vi "FP RT main.vi"() -> ()   [LabVIEW 2014]
uses:
  <vilib>/userdefined/High Color/IMAQdx.ctl
  <vilib>/myRIO/Instrument Drivers/Onboard IO/PWM/typedefs/PWM Reference.ctl
  <vilib>/myRIO/Common/Instrument Driver Framework/Utilities/typedefs/myRIO Generic Hardware Reference.ctl
  <vilib>/myRIO/Common/Instrument Driver Framework/Utilities/typedefs/Hardware Version Enum.ctl
  <vilib>/myRIO/Common/Instrument Driver Framework/Utilities/typedefs/myRIO v1.0 Reference.ctl
  <vilib>/myRIO/Common/Instrument Driver Framework/Utilities/typedefs/Generic FPGA Reference.ctl
  <vilib>/myRIO/Common/Instrument Driver Framework/myRIO v1.0/PWM/typedefs/PWM Channels Enum.ctl
  <vilib>/myRIO/Instrument Drivers/Onboard IO/PWM/typedefs/PWM Configuration.ctl
  <vilib>/userdefined/High Color/nirio_resource_hc.ctl
  <vilib>/myRIO/Instrument Drivers/Onboard IO/DIO/typedefs/DIO Reference.ctl
  <vilib>/myRIO/Common/Instrument Driver Framework/myRIO v1.0/DIO/typedefs/DIO Channels List.ctl
  <vilib>/myRIO/Common/Instrument Driver Framework/myRIO v1.0/DIO/typedefs/DIO Channels Enum.ctl
  <vilib>/myRIO/Instrument Drivers/Onboard IO/AI/typedefs/AI Reference.ctl
  <vilib>/myRIO/Common/Instrument Driver Framework/myRIO v1.0/AI/typedefs/AI Channels List.ctl
  <vilib>/myRIO/Common/Instrument Driver Framework/myRIO v1.0/AI/typedefs/AI Channels Enum.ctl
  <vilib>/myRIO/Common/Instrument Driver Framework/Utilities/typedefs/Analog Scaling Constants List.ctl
  <vilib>/myRIO/Common/Instrument Driver Framework/Utilities/typedefs/Analog Scaling Constants.ctl
  <vilib>/myRIO/Common/Instrument Driver Framework/myRIO v1.0/PWM/vis/myRIO v1.1 Open PWM.vi
  <vilib>/myRIO/Common/Instrument Driver Framework/myRIO v1.0/DIO/vis/myRIO v1.1 Open DIO.vi
  <vilib>/myRIO/Common/Instrument Driver Framework/myRIO v1.0/AI/vis/myRIO v1.1 Open AI.vi
  <vilib>/myRIO/Common/Instrument Driver Framework/Utilities/vis/Validate Channels.vi
  <vilib>/myRIO/Common/Instrument Driver Framework/myRIO v1.0/PWM/vis/myRIO v1.0 Reserve PWM.vi
  <vilib>/myRIO/Common/Instrument Driver Framework/myRIO v1.0/DIO/vis/myRIO v1.0 Reserve DIO.vi
  <vilib>/myRIO/Common/Instrument Driver Framework/myRIO v1.0/AI/vis/myRIO v1.0 Reserve AI.vi
  <vilib>/myRIO/Common/Instrument Driver Framework/myRIO v1.0/PWM/vis/myRIO v1.0 Build MUX Configuration PWM.vi
  <vilib>/myRIO/Common/Instrument Driver Framework/myRIO v1.0/Resource Manager/vis/myRIO v1.0 Reserve Channel List.vi
  <vilib>/myRIO/Common/Instrument Driver Framework/myRIO v1.0/DIO/vis/myRIO v1.0 Build MUX Configuration DIO.vi
  <vilib>/myRIO/Common/Instrument Driver Framework/myRIO v1.0/AI/vis/myRIO v1.0 Build MUX Configuration AI.vi
  <vilib>/myRIO/Common/Instrument Driver Framework/myRIO v1.0/Resource Manager/vis/myRIO v1.0 Create Configuration List.vi
  <vilib>/myRIO/Common/Instrument Driver Framework/myRIO v1.0/Resource Manager/vis/myRIO v1.0 Reserve Channel.vi
  <vilib>/myRIO/Common/Instrument Driver Framework/myRIO v1.0/Resource Manager/vis/myRIO v1.0 Unreserve Channel.vi
  <vilib>/myRIO/Common/Instrument Driver Framework/myRIO v1.0/Resource Manager/vis/myRIO v1.0 Build Mutex Name.vi
  <vilib>/Utility/VariantDataType/GetNumericInfo.vi
  <vilib>/Utility/error.llb/Error Cluster From Error Code.vi
  <vilib>/myRIO/Common/Instrument Driver Framework/myRIO v1.0/myRIO v1.1 Open.vi
  <vilib>/myRIO/Common/Instrument Driver Framework/myRIO v1.0/AI/vis/myRIO v1.0 Get Scaling Constants AI.vi
  <vilib>/myRIO/Common/Instrument Driver Framework/Utilities/vis/IO Manager.vi
  <vilib>/myRIO/Common/Instrument Driver Framework/Utilities/vis/Configuration Manager.vi
  <vilib>/myRIO/Common/Instrument Driver Framework/myRIO v1.0/myRIO v1.0 Close.vi
  <vilib>/myRIO/Common/Instrument Driver Framework/myRIO v1.0/Resource Manager/vis/myRIO v1.0 Configure IO.vi
  <vilib>/myRIO/Instrument Drivers/Onboard IO/AI/vis/myRIO AI Open.xnode
  <vilib>/myRIO/Instrument Drivers/Onboard IO/DIO/vis/myRIO DIO Open.xnode
  <vilib>/myRIO/Instrument Drivers/Onboard IO/PWM/vis/myRIO PWM Open.xnode
  <vilib>/vision/driver/NI_Vision_Acquisition_Software.lvlib
  <vilib>/myRIO/Instrument Drivers/Onboard IO/AI/AI.lvlib
  <vilib>/myRIO/Instrument Drivers/Onboard IO/DIO/DIO.lvlib
  <vilib>/myRIO/Instrument Drivers/Onboard IO/PWM/PWM.lvlib
panel:
  in  "Tab Control":T1(tab)
  out "GLED":bool
  out "BLED":bool
  out "RLED":bool
  out "BW Image":T2(plugin-control)
  in  "stop":bool
  out "Midbrain?":bool
  out "Rudder":dbl(knob) min=-45.0 max=45.0 step=1.0 scale=-45.0..45.0
  out "Speed":dbl(knob) min=-9.0 max=9.0 step=1.0 scale=-50.0..50.0
  out "Hindbrain?":bool
  out "Forebrain?":bool
  out "Battery Dead?":bool
  out "Complete?":bool=TRUE
  out "Arbiter Graph":cluster{dbl, dbl, dbl[]}(graph)
  in  "Session In":T3="cam0"
  out "Color Image":T2(plugin-control)
  out "Nb Circles":i32
  out "UDP Time Out?":bool
  in  "Tug letter":string="G"
  in  "Run?":bool
  in  "MSpeed":dbl(slide) scale=-50.0..50.0 scale format="%#.1g"
  in  "MHeading":dbl(slide) scale=-180.0..180.0 scale format="%_1f"
  in  "Manual?":bool
  out "Camera Data":T4(array[cluster])
  out "Boat Status":T5={"GPS"={"X pos"=0, "Y pos"=0, "Heading"=0.0}, "IR Sensors"=[{"Name"="Bow", "Angle"=0.0, "Distance"=0.0}], "MOT BAT"=7.2, "RIO BAT"=7.2}
  out "GPS?":bool
  out "Act Com":T6
  out "Forebrain ACT":dbl[](array[numeric])
  out "IR Sensors":T7(array[cluster])
  out "GPS":cluster{"X pos":i32, "Y pos":i32, "Heading":dbl}
  out "RED LED":bool
  out "GREEN LED":bool
  out "BLUE LED":bool
  in  "MDF":T8(array[cluster])=[{"Type"=enum."Start", "X"=250, "Y"=250, "Speed"=0, "Behaviors"=enum."Open Water Transit"}, {"Type"=enum."Waypoint", "X"=400, "Y"=100, "Speed"=20, "Behaviors"=enum."P-Wall Follow"}, {"Type"=enum."Waypoint", "X"=250, "Y"=250, "Speed"=20, "Behaviors"=enum."Open Water Transit"}, {"Type"=enum."Waypoint", "X"=250, "Y"=400, "Speed"=20, "Behaviors"=enum."Open Water Transit"}, {"Type"=enum."Waypoint", "X"=100, "Y"=400, "Speed"=20, "Behaviors"=enum."Open Water Transit"}, {"Type"=enum."End", "X"=250, "Y"=250, "Speed"=0, "Behaviors"=enum."Open Water Transit"}]
  out "Invalid Pos?":bool
  out "error out":errorcluster
  out "Forebrain Comd":T9
  out "Debug IR \nRaw Readings":T7(array[cluster])
  out "size(s)":i32
  out "MDF Active":T8(array[cluster])
  # "BEHAVIOR LIGHTS"
  # "To start the Tug, press the \">\" key in the tool bar.\n\nPress the Run? control to start the Mission.\n\nWhen complete the Complete? indicator will light.\n\nIf the Run? is not pressed again, the mission will start again.\n\nAlways press the STOP button to end the operation!!!!!!!!!!!!!"
  # "Press the Manual? button to control\nthe Tug from the sliders"
  # "Stuck indicates that\nthe boat is not moving."
  # "Enter the Letter\nof  your Tug"
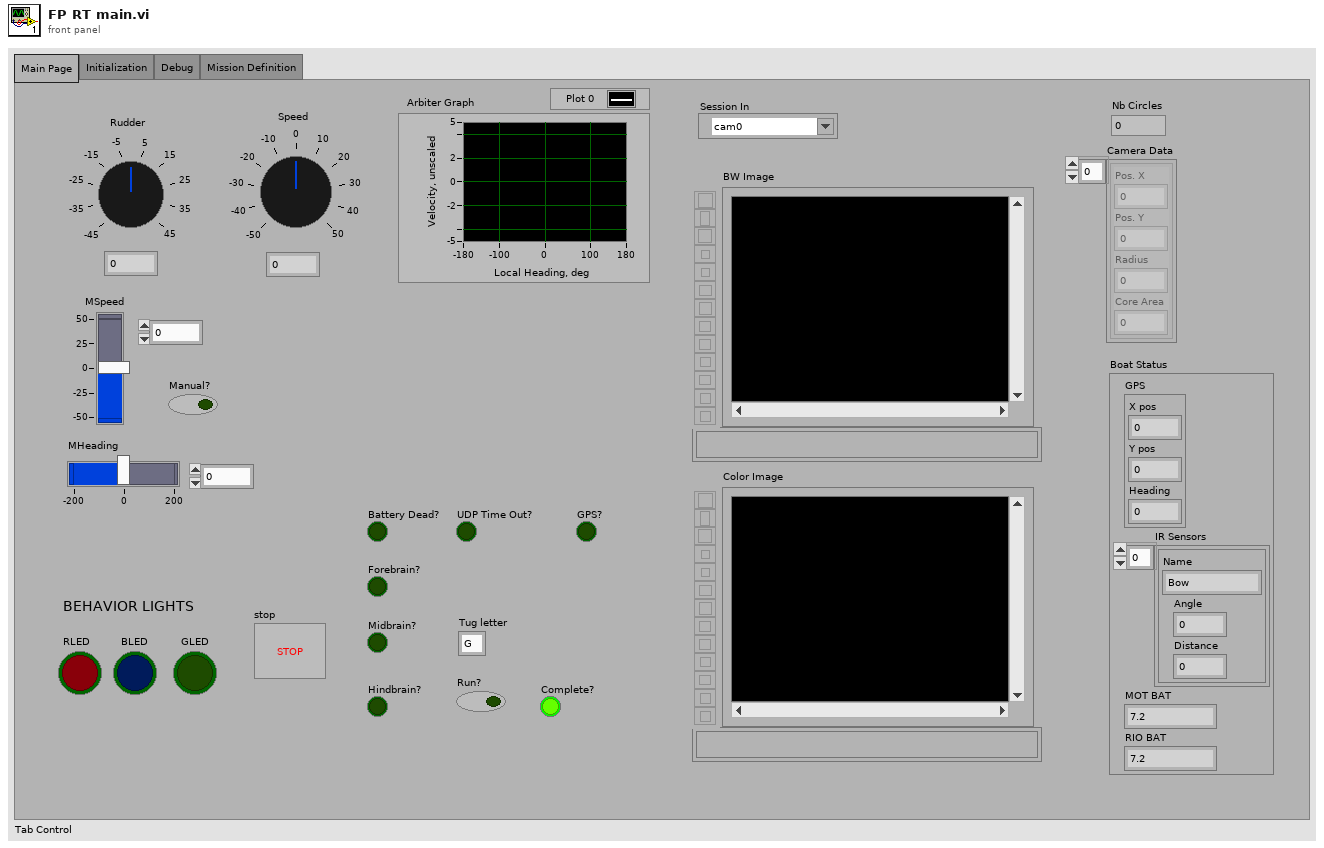
[diagram p1: front panel]
types:
  T1 = enum32{"Main Page", "Initialization", "Debug", "Mission Definition"}
  T2 = typedef "IMAQ Image.ctl" = refnum<image>
  T3 = typedef "IMAQdx.ctl" = refnum<k21>
  T4 = cluster{"Pos. X":i32, "Pos. Y":i32, "Radius":i32, "Core Area":i32}[]
  T5 = cluster{"GPS":cluster{"X pos":i32, "Y pos":i32, "Heading":dbl}, "IR Sensors":cluster{"Name":string, "Angle":dbl, "Distance":dbl}[], "MOT BAT":dbl, "RIO BAT":dbl}
  T6 = cluster{"Desired Local\nHeading":dbl, "Desired\nSpeed":dbl}
  T7 = cluster{"Name":string, "Angle":dbl, "Distance":dbl}[]
  T8 = cluster{"Type":enum16{"Start", "Waypoint", "End"}, "X":i32, "Y":i32, "Speed":i32, "Behaviors":enum16{"Open Water Transit", "P-Wall Follow", "S-Wall Follow", "Dock"}}[]
  T9 = cluster{"Behaviors":enum16{"Open Water Transit", "P-Wall Follow", "S-Wall Follow", "Dock"}, "Behavior\nVelocity":dbl}
  T10 = typedef "nirio_resource_hc.ctl" = tag
  T11 = typedef "Hardware Version Enum.ctl" = enum16{"Unknown", "myRIO-1900", "myRIO-1950"}
  T12 = typedef "Image Type" = u32
  T13 = enum16{"Open Water Transit", "P-Wall Follow", "S-Wall Follow", "Dock"}
  T14 = typedef "PWM.lvlib/PWM Reference.ctl" = cluster{"myRIO Reference":T15, "PWM Channels Enum":T18, "PWM Configuration":T19}
  T15 = typedef "myRIO Generic Hardware Reference.ctl" = cluster{"myRIO Model":T11, "myRIO Hardware Reference":T16}
  T16 = typedef "myRIO v1.0 Reference.ctl" = cluster{"Generic FPGA Reference":T17, "Allow multiple opens":bool}
  T17 = typedef "Generic FPGA Reference.ctl" = refnum<k20>
  T18 = typedef "PWM Channels Enum.ctl" = enum16{"Not Connected", "C/PWM0", "C/PWM1", "A/PWM0", "A/PWM1", "A/PWM2", "B/PWM0", "B/PWM1", "B/PWM2"}
  T19 = typedef "PWM.lvlib/PWM Configuration.ctl" = cluster{"Frequency":dbl, "Duty Cycle":dbl}
  T20 = typedef "DIO.lvlib/DIO Reference.ctl" = cluster{"myRIO Reference":T15, "DIO Channels List":T21}
  T21 = typedef "DIO Channels List.ctl" = T22[]
  T22 = typedef "DIO Channels Enum.ctl" = enum16{"Not Connected", "C/DIO0", "C/DIO1", "C/DIO2", "C/DIO3", "C/DIO4", "C/DIO5", "C/DIO6", "C/DIO7", "A/DIO0", "A/DIO1", "A/DIO2", "A/DIO3", "A/DIO4", "A/DIO5", "A/DIO6", "A/DIO7", "A/DIO8", "A/DIO9", "A/DIO10", "A/DIO11", "A/DIO12", "A/DIO13", "A/DIO14", "A/DIO15", "B/DIO0", "B/DIO1", "B/DIO2", "B/DIO3", "B/DIO4", "B/DIO5", "B/DIO6", "B/DIO7", "B/DIO8", "B/DIO9", "B/DIO10", "B/DIO11", "B/DIO12", "B/DIO13", "B/DIO14", "B/DIO15", "LED0", "LED1", "LED2", "LED3", "Button0"}
  T23 = typedef "AI.lvlib/AI Reference.ctl" = cluster{"myRIO Reference":T15, "AI Channels List":T24, "AI Scaling Constants List":T26}
  T24 = typedef "AI Channels List.ctl" = T25[]
  T25 = typedef "AI Channels Enum.ctl" = enum16{"Not Connected", "AudioIn/Left", "AudioIn/Right", "C/AI0", "C/AI1", "A/AI0", "A/AI1", "A/AI2", "A/AI3", "B/AI0", "B/AI1", "B/AI2", "B/AI3"}
  T26 = typedef "Analog Scaling Constants List.ctl" = T27[]
  T27 = typedef "Analog Scaling Constants.ctl" = cluster{"LSB Weight (Volts)":dbl, "Offset (Volts)":dbl, "Signed?":bool}
  T28 = cluster{"Obs Avoid Array":dbl[], "P-Wall Array":dbl[], "S-Wall Array":dbl[], "Unstuck Array":dbl[]}
  T29 = cluster{"regular expression":string, i32, i32, i32}
  T30 = cluster{"Behaviors":enum16{"Open Water Transit", "P-Wall Follow", "S-Wall Follow", "Dock"}, dbl}
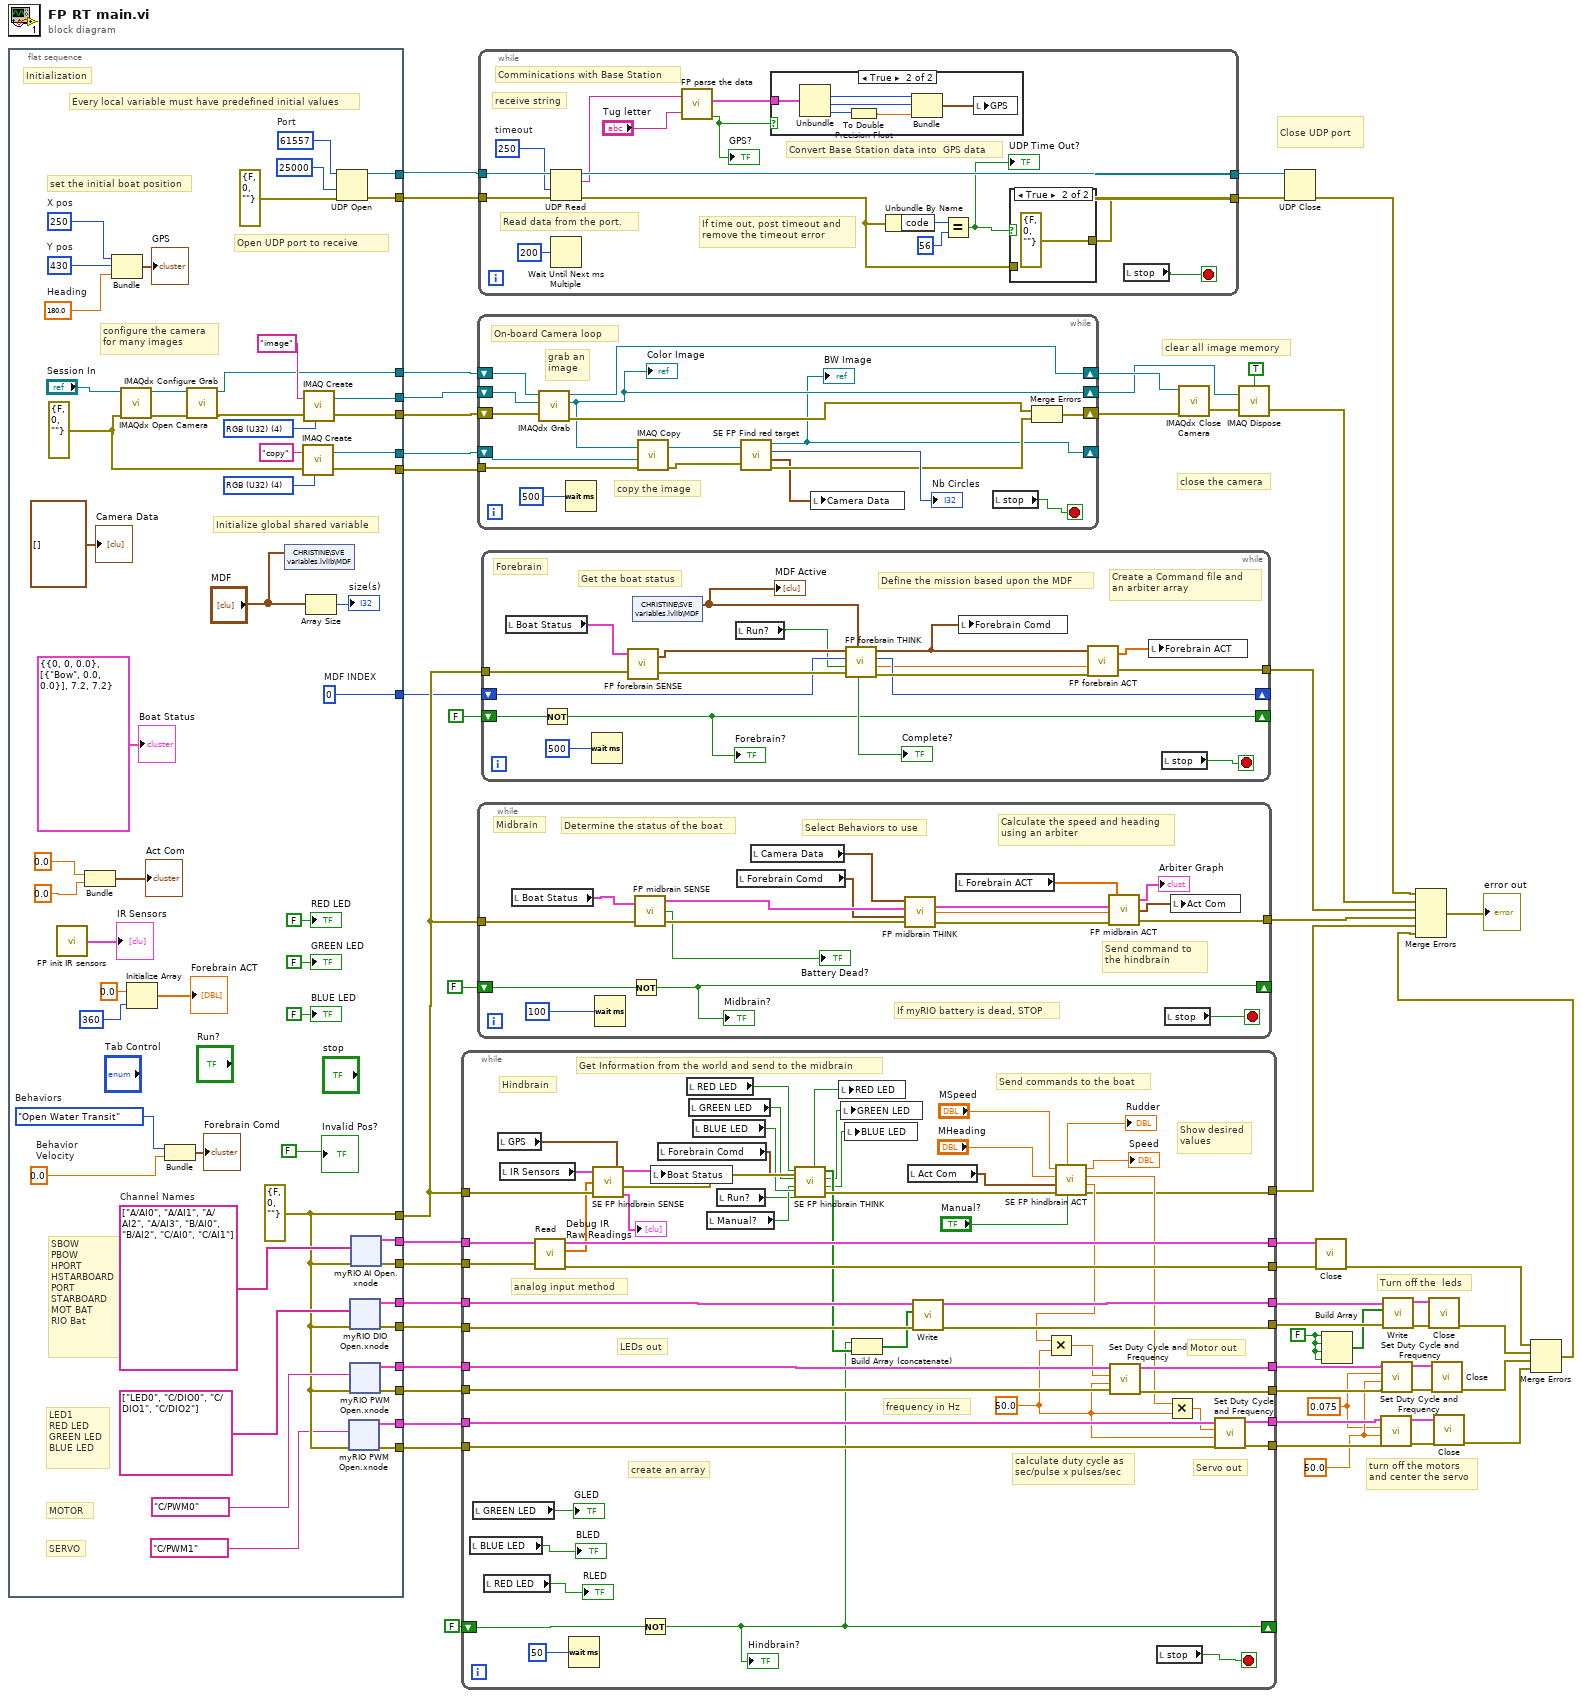
[diagram p0: block diagram]
diagram:
  w2 = 0.075
  w1 = FALSE
  w3 = 50.0
  # "Turn off the  leds"
  # "turn off the motors\nand center the servo"
  # "Close UDP port"
  # "clear all image memory"
  # "close the camera"
  n1 = flat-sequence {
    tunnel: [w68] -> w51
    tunnel: [w103] -> w48
    tunnel: [w94] -> w47
    tunnel: [w93] -> w46
    tunnel: [w92] -> w45
    tunnel: [w88] -> w38
    tunnel: [w87] -> w39
    tunnel: [w83] -> w33
    tunnel: [w82] -> w34
    tunnel: [w76] -> w31
    tunnel: [w75] -> w30
    tunnel: [w73] -> w26
    tunnel: [w72] -> w27
    tunnel: [w70] -> w25
    tunnel: [w69] -> w24
    tunnel: [w66] -> w23
    tunnel: [w65] -> w22
    frame #0 {
      w77 = tag[] ["A/AI0", "A/AI1", "A/AI2", "A/AI3", "B/AI0", "B/AI2", "C/AI0", "C/AI1"]  # Channel Names
      w79 = 430  # Y pos
      w80 = 250  # X pos
      w81 = 180.0  # Heading
      w86 = u16 61557  # Port
      w91 = T12 4 items=["Grayscale (U8)", "Grayscale (I16)", "Grayscale (SGL)", "Complex (CSG)", "RGB (U32)", "HSL (U32)", "RGB (U64)", "Grayscale (U16)"] ("Image Type")
      w89 = errorcluster {"status"=FALSE, "code"=0, "source"=""} ("error in")
      w99 = T12 4 items=["Grayscale (U8)", "Grayscale (I16)", "Grayscale (SGL)", "Complex (CSG)", "RGB (U32)", "HSL (U32)", "RGB (U64)", "Grayscale (U16)"] ("Image Type")
      w68 = errorcluster {"status"=FALSE, "code"=0, "source"=""} ("error out")
      w103 = 0  # MDF INDEX
      w107 = 0.0  # Behavior Velocity
      w102 = T13."Open Water Transit"  # Behaviors
      # "Initialize global shared variable"
      # "LED1\nRED LED\nGREEN LED\nBLUE LED"
      # "SERVO"
      # "MOTOR"
      # "SBOW\nPBOW\nHPORT\nHSTARBOARD\nPORT\nSTARBOARD\nMOT BAT\nRIO Bat"
      # "set the initial boat position"
      # "Open UDP port to receive"
      # "configure the camera\nfor many images"
      # "Every local variable must have predefined initial values"
      # "Initialization"
      n2 = call "FP init IR sensors.vi"() -> ("IR Sensors"=→"IR Sensors":T7)  [unwired: 1 in]
      n3 = Bundle(0.0, 0.0) -> (→"Act Com":cluster{dbl, dbl})  [unwired: 1 in]
      n4 = Bundle("X pos"=w80, "Y pos"=w79, "Heading"=w81) -> (→"GPS":cluster{"X pos":i32, "Y pos":i32, "Heading":dbl})  [unwired: 1 in]
      n5 = call <vilib>:"IMAQdx Open Camera.vi"("error in"=w89, "Session In"="Session In") -> ("error out"=w96:errorcluster, "Session Out"=w95:T3)  [unwired: 1 in, 7 out]
      n6 = Initialize Array(0.0 ("element"), 360 ("dimension size")) -> (→"Forebrain ACT":dbl[])
      n7 = Bundle("Behaviors"=w102, "Behavior\nVelocity"=w107) -> (→"Forebrain Comd":T9)  [unwired: 1 in]
      n8 = call <vilib>:"IMAQdx Configure Grab.vi"("error in"=w96, "Session In"=w95) -> ("error out"=w100:errorcluster, "Session Out"=w92:T3)  [unwired: 8 out]
      n9 = shared-variable "CHRISTINE\\SVE variables.lvlib\\MDF"("MDF") -> ()  [unwired: 1 in, 1 out]
      n10 = call "IMAQ Create"("Image Name"="copy", "Image Type"=w91, "error in (no error)"=w89) -> ("New Image"=w87:T2, "error out"=w88:errorcluster)  [unwired: 2 in]
      n11 = call "IMAQ Create"("Image Name"="image", "Image Type"=w99, "error in (no error)"=w100) -> ("New Image"=w93:T2, "error out"=w94:errorcluster)  [unwired: 1 in, 1 out]
      n12 = Array Size(array="MDF") -> (size(s)=→"size(s)":i32)
      n13 = UDP Open(8:errorcluster {"status"=FALSE, "code"=0, "source"=""} ("error in"), 9:25000 ("timeout ms (25000)"), 11:w86) -> (port=w83:refnum<k16>, 0:w82:errorcluster)  [unwired: 2 in, 1 out]
      n14 = xnode "myRIO PWM Open.xnode"("error in (no error)"=w68, "Channel Name"=tag "C/PWM1") -> ("error out"=w66:errorcluster, "PWM Ref Out"=w65:T14)  [unwired: 1 in]
      n15 = xnode "myRIO DIO Open.xnode"("error in (no error)"=w68, "Channel Names"=tag[] ["LED0", "C/DIO0", "C/DIO1", "C/DIO2"]) -> ("error out"=w73:errorcluster, "DIO Ref Out"=w72:T20)  [unwired: 1 in]
      n16 = xnode "myRIO PWM Open.xnode"("error in (no error)"=w68, "Channel Name"=tag "C/PWM0") -> ("error out"=w70:errorcluster, "PWM Ref Out"=w69:T14)  [unwired: 1 in]
      n17 = xnode "myRIO AI Open.xnode"("error in (no error)"=w68, "Channel Names"=w77) -> ("error out"=w76:errorcluster, "AI Ref Out"=w75:T23)  [unwired: 1 in]
      "Invalid Pos?" <- FALSE
      "RED LED" <- FALSE ("RED LED")
      "GREEN LED" <- FALSE ("GREEN LED")
      "BLUE LED" <- FALSE ("WHITE LED")
      "Camera Data" <- T4 [] ("Camera Data")
      "Boat Status" <- T5 {"GPS"={"X pos"=0, "Y pos"=0, "Heading"=0.0}, "IR Sensors"=[{"Name"="Bow", "Angle"=0.0, "Distance"=0.0}], "MOT BAT"=7.2, "RIO BAT"=7.2} ("Boat Status 2")
    }
  }
  n18 = while {
    tunnel: w51 -> [w228]
    tunnel: [w202] -> w55
    shift-right: [w190] -> _
    shift-left: FALSE -> [w217]
    tunnel: w31 -> [w225]
    tunnel: w30 -> [w224]
    tunnel: [w223] -> w29
    tunnel: [w222] -> w28
    tunnel: w27 -> [w220]
    tunnel: w26 -> [w221]
    tunnel: [w219] -> w8
    tunnel: [w218] -> w5
    tunnel: w25 -> [w215]
    tunnel: w24 -> [w216]
    tunnel: [w214] -> w17
    tunnel: [w213] -> w14
    tunnel: w23 -> [w212]
    tunnel: [w211] -> w21
    tunnel: w22 -> [w210]
    tunnel: [w209] -> w19
    stop <- w230 stop-if-true
    w204 = 50.0
    # "create an array"
    # "frequency in Hz"
    # "calculate duty cycle as\nsec/pulse x pulses/sec"
    # "Show desired\nvalues"
    # "Motor out"
    # "Servo out"
    # "LEDs out"
    # "analog input method"
    # "Send commands to the boat"
    # "Get Information from the world and send to the midbrain"
    # "Hindbrain"
    n19 = local read "BLUE LED"() -> (→"BLED":bool)
    n20 = local read "GREEN LED"() -> (→"GLED":bool)
    n21 = local read "RED LED"() -> (→"RLED":bool)
    n22 = local read "GPS"() -> (w226:cluster{"X pos":i32, "Y pos":i32, "Heading":dbl})
    n23 = local read "IR Sensors"() -> (w188:T7)
    n24 = call <vilib>:"Read.vi"("error in (no error)"=w225, "AI Ref In"=w224) -> ("error out"=w223:errorcluster, "Values"=w208:dbl[], "AI Ref Out"=w222:T23)  [unwired: 7 in]
    n25 = Wait (ms)(milliseconds to wait=u32 50) -> ()  [unwired: 1 out]
    n26 = call "SE FP hindbrain SENSE.vi"("IR Sensors"=w188, "Analog Input Values"=w208, "error in"=w228, "GPS"=w226) -> ("Boat Status"=w189:T5, "error out"=w227:errorcluster, "IR Sensors 2"=→"Debug IR \nRaw Readings":T7)
    n27 = Not(x=w217) -> (.not. x?=w190:bool)
    "Hindbrain?" <- w190
    n28 = local write "Boat Status"(w189) -> ()
    n29 = local read "Forebrain Comd"() -> (w187:T9)
    n30 = local read "RED LED"() -> (w193:bool)
    n31 = local read "GREEN LED"() -> (w192:bool)
    n32 = local read "BLUE LED"() -> (w191:bool)
    n33 = local read "Manual?"() -> (w183:bool)
    n34 = local read "Run?"() -> (w178:bool)
    n35 = call "SE FP hindbrain THINK.vi"("error in"=w227, "BLUE LED"=w191, "Forebrain Comd"=w187, "RUN?"=w178, "MANUAL"=w183, "GREEN LED"=w192, "RED LED"=w193) -> ("error out"=w202:errorcluster, "BLUE LED OUT"=w184:bool, "GREEN LED OUT"=w185:bool, "LED array"=w195:bool[], "RED LED OUT"=w186:bool)
    n36 = local write "RED LED"(w186) -> ()
    n37 = local write "GREEN LED"(w185) -> ()
    n38 = local write "BLUE LED"(w184) -> ()
    n39 = Build Array (concatenate)(w190, w195) -> (w194:bool[])
    n40 = local read "Act Com"() -> (w199:T6)
    n41 = call <vilib>:"Write.vi"("error in (no error)"=w221, "Values"=w194, "DIO Ref In"=w220) -> ("error out"=w219:errorcluster, "DIO Ref Out"=w218:T20)  [unwired: 6 in]
    n42 = call "SE FP hindbrain ACT.vi"("Manual?"="Manual?", "error in"=w202, "Act Com"=w199, "MHeading"="MHeading", "MSpeed"="MSpeed") -> ("Speed"=w207:dbl, "Rudder"=w205:dbl, "Desired\nSpeed"=→"Speed":dbl, "Desired \nRudder"=→"Rudder":dbl)  [unwired: 1 out]
    n43 = Multiply(x=w207, y=w204) -> (x*y=w206:dbl)
    n44 = call <vilib>:"Set Duty Cycle and Frequency.vi"("error in (no error)"=w215, "Frequency [Hz]"=w204, "Duty Cycle"=w206, "PWM Ref In"=w216) -> ("error out"=w214:errorcluster, "PWM Ref Out"=w213:T14)  [unwired: 5 in]
    n45 = local read "stop"() -> (w230:bool)
    n46 = Multiply(x=w205, y=w204) -> (x*y=w203:dbl)
    n47 = call <vilib>:"Set Duty Cycle and Frequency.vi"("error in (no error)"=w212, "Frequency [Hz]"=w204, "Duty Cycle"=w203, "PWM Ref In"=w210) -> ("error out"=w211:errorcluster, "PWM Ref Out"=w209:T14)  [unwired: 5 in]
  }
  n48 = while {
    shift-right: [w234] -> w43
    shift-left: w47 -> [w246]
    shift-right: [w233] -> w41
    shift-left: w46 -> [w245]
    shift-right: [w238] -> w42
    shift-left: w45 -> [w244]
    tunnel: w38 -> [w242]
    shift-right: [w232] -> _
    shift-left: w39 -> [w241]
    stop <- w247 stop-if-true
    # "grab an\nimage"
    # "copy the image"
    # "On-board Camera loop"
    n49 = call <vilib>:"IMAQdx Grab.vi"("error in"=w246, "Image In"=w245, "Session In"=w244) -> ("error out"=w235:errorcluster, "Image Out"=w233:T2, "Session Out"=w238:T3)  [unwired: 5 in, 1 out]
    "Color Image" <- w233
    n50 = Wait (ms)(milliseconds to wait=u32 500) -> ()  [unwired: 1 out]
    n51 = call "IMAQ Copy"("error in (no error)"=w242, "Image Dst"=w241, "Image Src"=w233) -> ("error out"=w240:errorcluster, "Image Dst Out"=w239:T2)  [unwired: 3 in]
    n52 = call "SE FP Find red target.vi"("Image In"=w239, "error in (no error)"=w240) -> ("Image Dst Out"=w232:T2, "Nb Circles (Circle Detection 1)"=→"Nb Circles":i32, "Camera Data"=w231:T4, "error out"=w236:errorcluster)
    "BW Image" <- w232
    n53 = local write "Camera Data"(w231) -> ()
    n54 = local read "stop"() -> (w247:bool)
    n55 = Merge Errors(w235, w236) -> (w234:errorcluster)
  }
  n56 = while {
    shift-right: [w253] -> _
    shift-left: FALSE -> [w264]
    tunnel: w51 -> [w263]
    tunnel: [w257] -> w53
    stop <- w265 stop-if-true
    # "If myRIO battery is dead, STOP"
    # "Send command to \nthe hindbrain"
    # "Calculate the speed and heading\nusing an arbiter"
    # "Select Behaviors to use"
    # "Determine the status of the boat"
    # "Midbrain"
    n57 = local read "Boat Status"() -> (w248:T5)
    n58 = Wait (ms)(milliseconds to wait=u32 100) -> ()  [unwired: 1 out]
    n59 = Not(x=w264) -> (.not. x?=w253:bool)
    "Midbrain?" <- w253
    n60 = call "FP midbrain SENSE.vi"("Boat Status"=w248, "error in"=w263) -> ("IR Sensors"=w251:T7, "Battery\nDead?"=→"Battery Dead?":bool, "error out"=w261:errorcluster)
    n61 = local read "Forebrain Comd"() -> (w250:T9)
    n62 = local read "Camera Data"() -> (w249:T4)
    n63 = call "FP midbrain THINK.vi"("error in"=w261, "Forebrain Comd"=w250, "IR Sensors"=w251, "Camera Data"=w249) -> ("error out"=w260:errorcluster, "Behavior\nVelocity OUT"=w255:dbl, "Behavior arrays"=w258:T28)
    n64 = local read "Forebrain ACT"() -> (w256:dbl[])
    n65 = call "FP midbrain ACT.vi"("error in"=w260, "Behavior\nVelocity"=w255, "Behavior arrays"=w258, "Forebrain ACT"=w256) -> ("error out"=w257:errorcluster, "Act Com"=w262:T6, "Waveform Graph"=→"Arbiter Graph":cluster{dbl, dbl, dbl[]})
    n66 = local read "stop"() -> (w265:bool)
    n67 = local write "Act Com"(w262) -> ()
  }
  n68 = while {
    tunnel: w34 -> [w280]
    tunnel: w33 -> [w279]
    tunnel: [w278] -> w36
    tunnel: [w273] -> w35
    stop <- w270 stop-if-true
    w272 = 250  # timeout
    # "Convert Base Station data into  GPS data"
    # "Comminications with Base Station"
    # "receive string"
    # "If time out, post timeout and\nremove the timeout error"
    # "Read data from the port."
    n69 = UDP Read(connection ID=w279, timeout ms (25000)=w272, 8:w280) -> (data out=w267:string, error out=w274:errorcluster, 3:w278:refnum<k16>)  [unwired: 1 in, 2 out]
    n70 = Wait Until Next ms Multiple(millisecond multiple=u32 200) -> ()  [unwired: 1 out]
    n71 = call "FP parse the data.vi"("Nav String"=w267, "Tug"="Tug letter") -> ("Tug Location"=w268:T29, "Valid?"=w266:bool)  [unwired: 2 out]
    "GPS?" <- w266
    n72 = case shown="True" w266 {
      tunnel: w268 -> [_ w286]
      frame False {
      }
      frame True {
        n73 = Unbundle(w286) -> (w285:i32, w284:i32, w282:i32)  [unwired: 1 out]
        n74 = To Double Precision Float(number=w282) -> (double precision float=w283:dbl)
        n75 = Bundle(w285, w284, w283) -> (w281:cluster{i32, i32, dbl})  [unwired: 1 in]
        n76 = local write "GPS"(w281) -> ()
      }
    }
    n77 = Unbundle By Name(w274) -> ("code"=w277:i32)
    n78 = Equal?(x=w277, y=56) -> (x = y?=w275:bool)
    "UDP Time Out?" <- w275
    n79 = case shown="True" w275 {
      tunnel: [w287 errorcluster {"status"=FALSE, "code"=0, "source"=""} ("error out")] -> w273
      tunnel: w274 -> [w287 _]
      frame False {
      }
      frame True {
      }
    }
    n80 = local read "stop"() -> (w270:bool)
  }
  n81 = while {
    tunnel: w51 -> [w304]
    shift-right: [w292] -> _
    shift-left: FALSE -> [w293]
    tunnel: [w301] -> w49
    shift-right: [w297] -> _
    shift-left: w48 -> [w295]
    stop <- w305 stop-if-true
    # "Create a Command file and \nan arbiter array"
    # "Define the mission based upon the MDF"
    # "Get the boat status"
    # "Forebrain"
    n82 = local read "Boat Status"() -> (w299:T5)
    n83 = Not(x=w293) -> (.not. x?=w292:bool)
    "Forebrain?" <- w292
    n84 = Wait (ms)(milliseconds to wait=u32 500) -> ()  [unwired: 1 out]
    n85 = call "FP forebrain SENSE.vi"("error in"=w304, "Boat Status"=w299) -> ("error out"=w303:errorcluster, "GPS"=w298:cluster{"X pos":i32, "Y pos":i32, "Heading":dbl})  [unwired: 1 in]
    n86 = shared-variable "CHRISTINE\\SVE variables.lvlib\\MDF"() -> (w289:T8)  [unwired: 1 in, 1 out]
    "MDF Active" <- w289
    n87 = local read "Run?"() -> (w291:bool)
    n88 = call "FP forebrain THINK.vi"("MDF in"=w289, "error in"=w303, "Run?"=w291, "MDF index"=w295, "GPS"=w298) -> ("error out"=w302:errorcluster, "local Steering\nangle"=w296:dbl, "MDF Index out"=w297:i32, "Behaviors out"=w290:T30, "Complete?"=→"Complete?":bool)
    n89 = local write "Forebrain Comd"(w290) -> ()
    n90 = call "FP forebrain ACT.vi"("error in"=w302, "local Steering\nangle"=w296, "Behaviors in"=w290) -> ("error out"=w301:errorcluster, "Forebrain ACT"=w300:dbl[])
    n91 = local write "Forebrain ACT"(w300) -> ()
    n92 = local read "stop"() -> (w305:bool)
  }
  n93 = call <vilib>:"IMAQdx Close Camera.vi"("error in"=w43, "Session In"=w42) -> ("error out"=w44:errorcluster)  [unwired: 9 out]
  n94 = call "IMAQ Dispose"("All Images? (No)"=TRUE, "Image"=w41, "error in (no error)"=w44) -> ("error out"=w40:errorcluster)  [unwired: 3 out]
  n95 = UDP Close(connection ID=w36, 8:w35) -> (error out=w32:errorcluster)  [unwired: 1 out]
  n96 = call <vilib>:"Close.vi"("error in (no error)"=w29, "AI Ref In"=w28) -> ("error out"=w10:errorcluster)  [unwired: 9 in]
  n97 = Build Array(w1, w1, w1, w1) -> (w4:bool[])
  n98 = call <vilib>:"Set Duty Cycle and Frequency.vi"("error in (no error)"=w21, "Frequency [Hz]"=w3, "Duty Cycle"=w2, "PWM Ref In"=w19) -> ("error out"=w20:errorcluster, "PWM Ref Out"=w18:T14)  [unwired: 5 in]
  n99 = call <vilib>:"Set Duty Cycle and Frequency.vi"("error in (no error)"=w17, "Frequency [Hz]"=w3, "Duty Cycle"=w2, "PWM Ref In"=w14) -> ("error out"=w16:errorcluster, "PWM Ref Out"=w15:T14)  [unwired: 5 in]
  n100 = call <vilib>:"Write.vi"("error in (no error)"=w8, "Values"=w4, "DIO Ref In"=w5) -> ("error out"=w7:errorcluster, "DIO Ref Out"=w6:T20)  [unwired: 6 in]
  n101 = call <vilib>:"Close.vi"("error in (no error)"=w7, "DIO Ref In"=w6) -> ("error out"=w11:errorcluster)  [unwired: 9 in]
  n102 = call <vilib>:"Close.vi"("error in (no error)"=w16, "PWM Ref In"=w15) -> ("error out"=w12:errorcluster)  [unwired: 9 in]
  n103 = call <vilib>:"Close.vi"("error in (no error)"=w20, "PWM Ref In"=w18) -> ("error out"=w13:errorcluster)  [unwired: 9 in]
  n104 = Merge Errors(w10, w11, w12, w13) -> (w9:errorcluster)
  n105 = Merge Errors(w32, w40, w49, w53, w55, w9) -> (→"error out":errorcluster)
